vi "Panel Overide Com Settings.vi"() -> (4 "COM Port Out":refnum<visa-resource-name>="COM3", 6 "GEA2 HyperData Out":bool)   [LabVIEW 2012]
panel:
  in  "stop":bool
  in  "GEA2 HyperData":bool
  in  "COM Port":refnum<visa-resource-name>="COM3"
  # "Communication Settings"
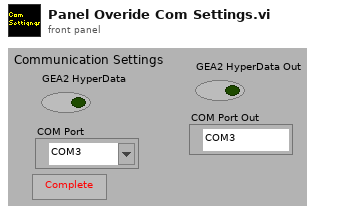
[diagram p1: front panel]
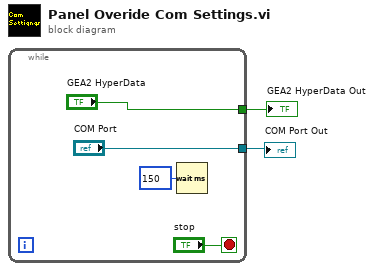
[diagram p0: block diagram]
diagram:
  n1 = while {
    tunnel: ["COM Port"] -> w2
    tunnel: ["GEA2 HyperData"] -> w1
    stop <- "stop" stop-if-true
    n2 = Wait (ms)(milliseconds to wait=u32 150) -> ()  [unwired: 1 out]
  }
  "GEA2 HyperData Out" <- w1
  "COM Port Out" <- w2
